vi "Feed-SISE-Probe-Graph.vi"(6 "Boolesch":bool, 7 "Numerisch":i32, 9 "Array 2":dbl[][](array[numeric]), 10 "Array":dbl[](array[numeric]), 11 "Start fit (% of rec. period)":dbl) -> (3 "Array 3":cluster{dbl[], dbl[]}[](array[cluster]))   [LabVIEW 2024]
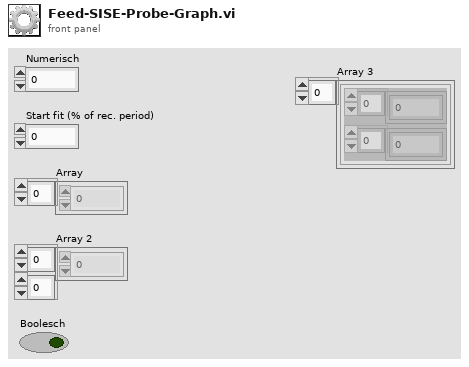
[diagram p1: front panel]
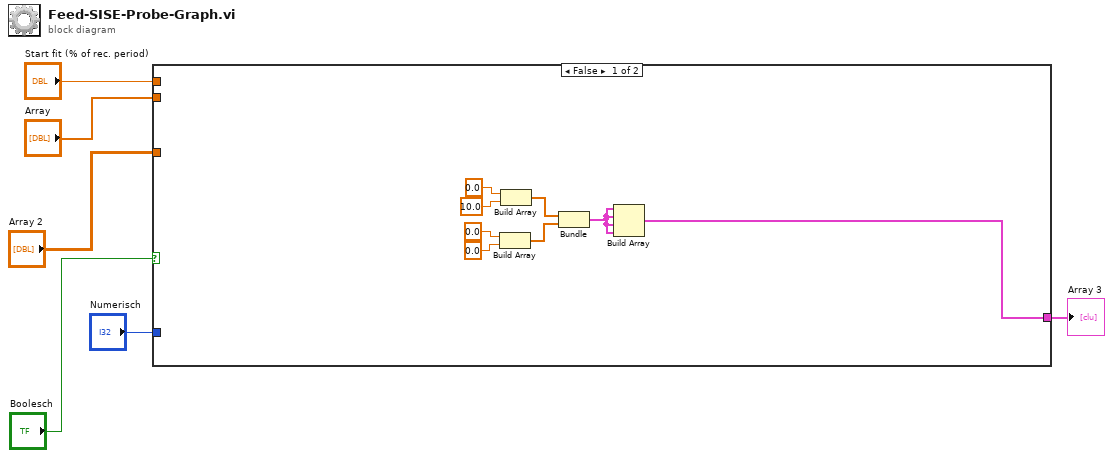
[diagram p0: block diagram]
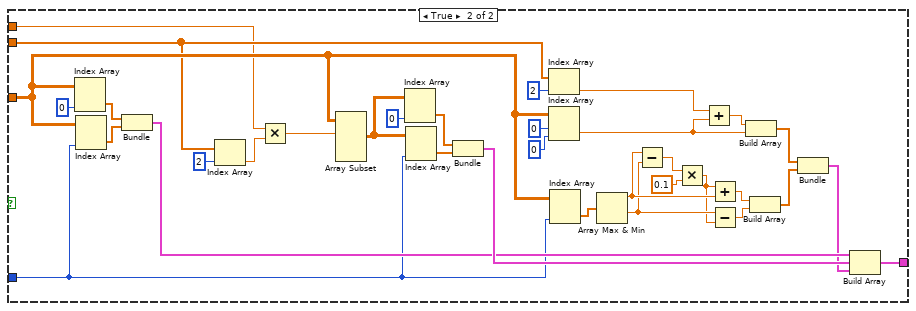
[diagram p2: hidden frame]
diagram:
  n1 = case shown="False" "Boolesch" {
    tunnel: [w7 w19] -> w1
    tunnel: "Array 2" -> [_ w18]
    tunnel: "Array" -> [_ w17]
    tunnel: "Start fit (% of rec. period)" -> [_ w16]
    tunnel: "Numerisch" -> [_ w15]
    frame False {
      n2 = Build Array(0.0, 0.0) -> (w9:dbl[])
      n3 = Build Array(0.0, 10.0) -> (w10:dbl[])
      n4 = Bundle(w10, w9) -> (w8:cluster{dbl[], dbl[]})  [unwired: 1 in]
      n5 = Build Array(w8, w8, w8, w8) -> (w7:cluster{dbl[], dbl[]}[])
    }
    frame True {
      n6 = Index Array(array=w18, index (col)=0 ("disabled index (col)")) -> (element=w46:dbl[])  [unwired: 1 in]
      n7 = Index Array(array=w18, index (col)=w15) -> (element=w47:dbl[])  [unwired: 1 in]
      n8 = Bundle("Array 2"=w46, "Array 2"=w47) -> (w39:cluster{"Array 2":dbl[], "Array 2":dbl[]})  [unwired: 1 in]
      n9 = Index Array(array=w17, index=2) -> (element=w21:dbl)
      n10 = Multiply(x=w16, y=w21) -> (x*y=w20:dbl)
      n11 = Array Subset(array=w18, index (row)=w20) -> (w41:dbl[][])  [unwired: 3 in]
      n12 = Index Array(array=w41, index (col)=0 ("disabled index (col)")) -> (element=w43:dbl[])  [unwired: 1 in]
      n13 = Index Array(array=w41, index (col)=w15) -> (element=w42:dbl[])  [unwired: 1 in]
      n14 = Bundle(w43, w42) -> (w40:cluster{dbl[], dbl[]})  [unwired: 1 in]
      n15 = Index Array(array=w17, index=2) -> (element=w23:dbl)
      n16 = Index Array(array=w18, index (row)=0, index (col)=0) -> (element=w24:dbl)
      n17 = Index Array(array=w18, index (col)=w15) -> (element=w37:dbl[])  [unwired: 1 in]
      n18 = Array Max & Min(array=w37) -> (max value=w32:dbl, min value=w31:dbl)  [unwired: 2 out]
      n19 = Subtract(x=w32, y=w31) -> (x-y=w35:dbl)
      n20 = Multiply(x=w35, y=0.1) -> (x*y=w29:dbl)
      n21 = Add(x=w23, y=w24) -> (x+y=w25:dbl)
      n22 = Add(x=w29, y=w32) -> (x+y=w33:dbl)
      n23 = Subtract(x=w31, y=w29) -> (x-y=w30:dbl)
      n24 = Build Array(w25, w24) -> (w22:dbl[])
      n25 = Build Array(w33, w30) -> (w38:dbl[])
      n26 = Bundle(w22, w38) -> (w36:cluster{dbl[], dbl[]})  [unwired: 1 in]
      n27 = Build Array(w39, w40, w36) -> (w19:cluster{"Array 2":dbl[], "Array 2":dbl[]}[])
    }
  }
  "Array 3" <- w1
